vi "Logout_from_webserver_with_idletime.vi"() -> ()   [LabVIEW 2017]
uses:
  Generic_Common/Webserver/html_report_cluster.ctl
  <vilib>/httpClient/LabVIEWHTTPClient.lvlib
panel:
  out "idle_time":string
  out "StatusCodeName":string
  out "Session id name":string
  out "logout_url":string
  out "ErrorCode_expected":string
  out "Logout : Header  debug purpose":string
  out "Logout : Body debug purpose":string
  out "Status_message":string
  out "Logo":u16(ring)
  out "Iteration_Indicator":dbl
  out "Error code recieved":i32
  out "POST_command":string
  out "Command_url":string
  out "Test case":string
  out "Global ini path":path
  out "Test status":picture
  out "Time elapsed for each iteration":string
  out "DelayBetweenIterations":string
  out "Total_Iterations":i32
  out "Global_Webserver_Report":string
  out "TestSuite":string
  out "Error Out":errorcluster
  out "Response time":u32[](graph)
  out "Header of reponse for debug pupose":string
  out "Response from the web server":string
  # "AUTOMATION TESTING WEB SERVICES"
  # "TESTING DETAILS FROM INI"
  # "RESPONSE FROM WEBSERVER"
  # "ms"
  # "Webserver \n1. Webserver is being tested in this test case where SC board of ultrasonic welding machine is connected to test PC \t\t  \nSC IP address: 192.168.2.101, url=https://192.168.2.101\t\t\t\t\t\t\t\t\t\t \t\t\t  \n2. Ports used on SC board are as below:\t\t\t\t\t\t\t\t\t\t\t\t\t\t\t\t\t\t\t\t\t  \n   - J103: (Ethernet0) This port connected to UI controller large screen HMI display\trestricted webservices in this port\t\t\t\t\t\t\t\t\t  \n  - J104: (Ethernet1) This port is connected to local area network for accessing the webpage and testing  webserver                                \n  - J112: SC Logs are taken from this port. TeraTerm is configured  to this port so that SC logs are displayed on the screen."
  # "ms"
  # "Debug purpose"
  # "RESPONSE TIME GRAPH"
  # "TESTING STATUS"
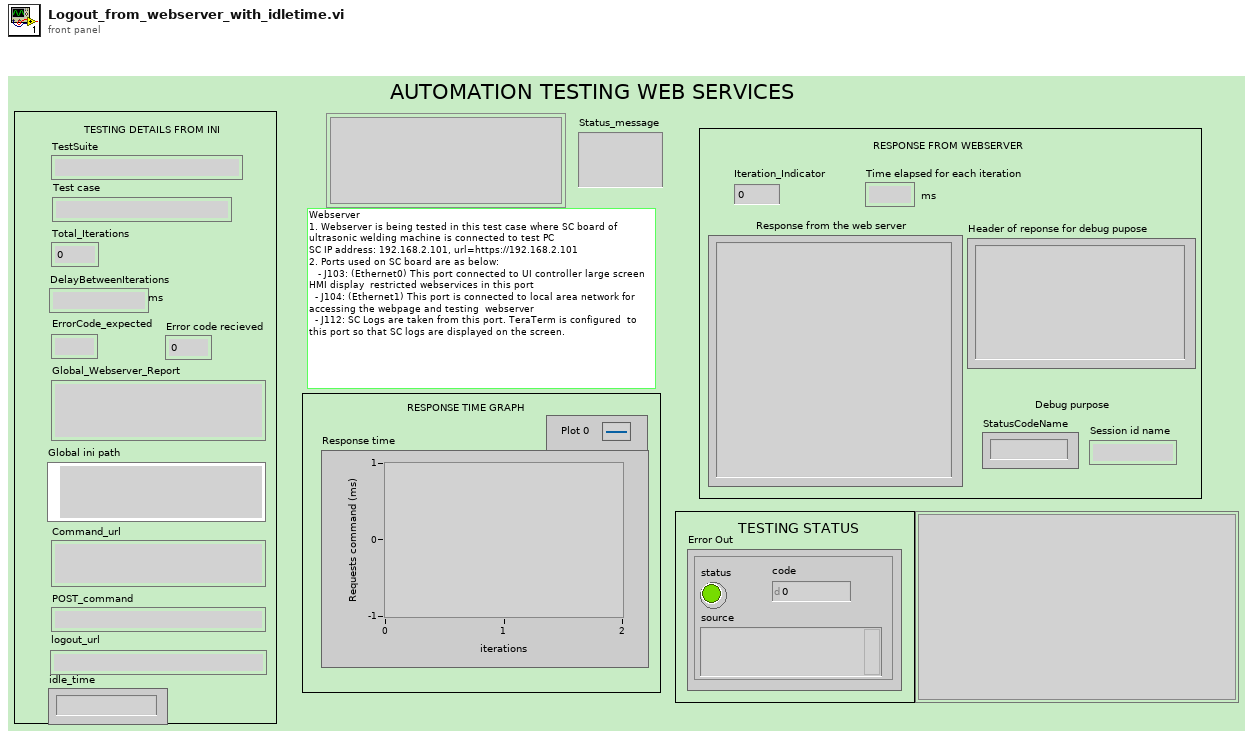
[diagram p1: front panel]
types:
  T1 = enum16{"open", "replace", "create", "open or create", "replace or create", "replace or create with confirmation"}
  T2 = enum8{"Enabled", "Disabled", "Disabled and Grayed Out"}
  T3 = cluster{"[0]":string, "[1]":string, "[2]":string, "[3]":string, "[4]":string, "[5]":string, "[6]":string, "[7]":string, "[8]":string}
  T4 = cluster{"login_url":string, "userid":string, "password":string, "idle_time":string, "command_url":string, "POST_command":string, "StatusCode_expected":string, "Iterations":string, "DelayBetweenIterations":string, "Timeout":string, "logout_url":string, "TestSuite":string, "key":string}
  T5 = cluster{"Server_IP_Address":string, "Server_Port_Number":string, "Sid":string, "StatusCodeName":string, "Global_Webserver_Report":string}
  T6 = typedef "html_report_cluster.ctl" = cluster{"Remarks":string, "Verdict":string, "Status Code":i32, "Status Description":string, "JazzDashboardLink":string, "ReprtPath":string, "Timestamp":string, "TestSuite":string, "TestCase":string, "Iterations":i64, "Time taken to execute  test in msec":string, "Delay Between Iterations":i64}
  T7 = typedef "LabVIEWHTTPClient.lvlib/ClientHandle.ctl" = refnum<k1>
  T8 = typedef "imagedata.ctl" = cluster{"image type":i32, "image depth":i32, "image":u8[], "mask":u8[], "colors":u32[], "Rectangle":cluster{"left":i16, "top":i16, "right":i16, "bottom":i16}}
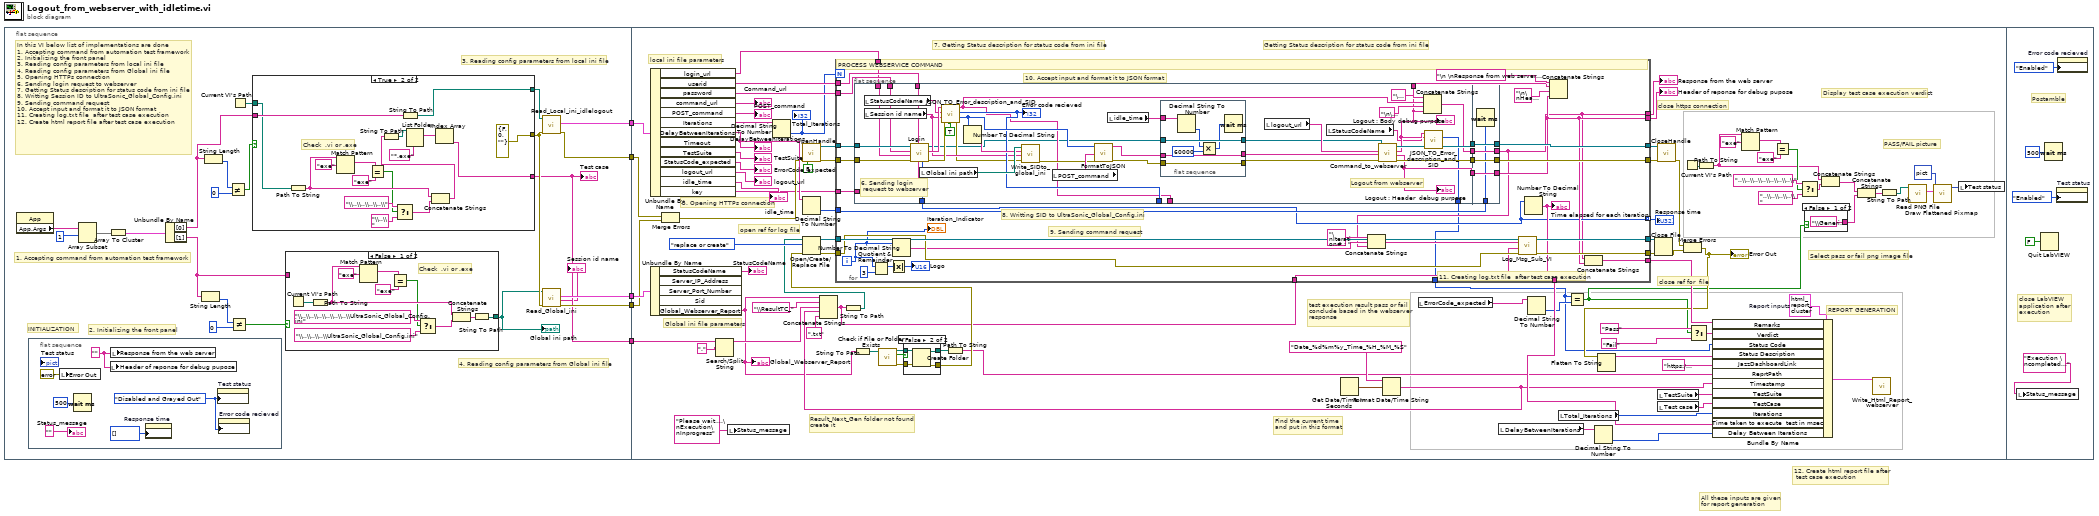
[diagram p0: block diagram]
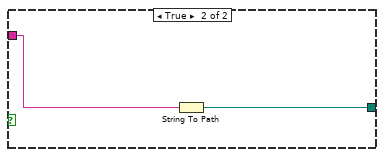
[diagram p2: hidden frame]
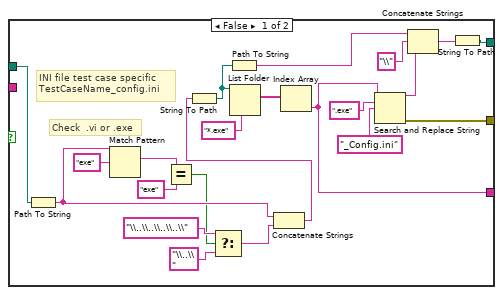
[diagram p3: hidden frame]
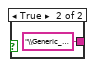
[diagram p5: hidden frame]
diagram:
  # "All these inputs are given \nfor report generation"
  # "12. Create html report file after\n test case execution"
  n1 = flat-sequence {
    tunnel: [w16] -> w5
    tunnel: [w19] -> w4
    tunnel: [w18] -> w3
    tunnel: [w17] -> w2
    tunnel: [w7] -> w1
    tunnel: w5 -> [w141]
    tunnel: w4 -> [w173]
    tunnel: w3 -> [w174]
    tunnel: w2 -> [w140]
    tunnel: w1 -> [w113]
    frame #0 {
      # "INITIALIZATION"
      # "4. Reading config parameters from Global ini file"
      # "3. Reading config parameters from local ini file"
      # "2. Initializing the front panel"
      # "1. Accepting command from automation test framework"
      # "In this VI below list of implementations are done\n1. Accepting command from automation test framework\n2. Initializing the front panel\n3. Reading config parameters from local ini file\n4. Reading config parameters from Global ini file\n5. Opening HTTPs connection\n6. Sending login request to webserver\n7. Getting Status description for status code from ini file\n8. Writting Session ID to UltraSonic_Global_Config.ini\n9. Sending command request\n10. Accept input and format it to JSON format\n11. Creating log.txt file  after test case execution\n12. Create html report file after test case execution"
      n2 = property class="App"() -> ("App.Args"=w21:string[])  [unwired: 2 in, 2 out]
      n3 = flat-sequence {
        frame #0 {
          w28 = T2."Disabled and Grayed Out" ("Disabled")
          w33 = ""
          n4 = local write "Error Out"(errorcluster {"status"=FALSE, "code"=0, "source"=""} ("error constant")) -> ()
          n5 = Wait (ms)(milliseconds to wait=u32 500) -> ()  [unwired: 1 out]
          n6 = local write "Header of reponse for debug pupose"(w33) -> ()
          n7 = local write "Response from the web server"(w33) -> ()
          n8 = property on="Response time" class="WFChart (strict)"("History Data"=u32[] []) -> ()  [unwired: 2 in, 2 out]
          n9 = property on="Test status" class="Pict"("DisabledEnum"=w28) -> ()  [unwired: 2 in, 2 out]
          n10 = property on="Error code recieved" class="DigNum (strict)"("DisabledEnum"=w28) -> ()  [unwired: 2 in, 2 out]
          "Status_message" <- ""
        }
      }
      n11 = Array Subset "Array Subset"(array=w21, index=1) -> (w22:string[])  [unwired: 1 in]
      n12 = Array To Cluster(array=w22) -> (cluster=w23:T3)
      n13 = Unbundle By Name "Unbundle By Name"(w23) -> ("[0]"=w15:string, "[1]"=w10:string)
      n14 = String Length(string=w10) -> (length=w27:i32)
      n15 = String Length(string=w15) -> (length=w24:i32)
      n16 = Not Equal?(x=w24, y=0) -> (x != y?=w13:bool)
      n17 = Not Equal?(x=w27, y=0) -> (x != y?=w11:bool)
      n18 = Current VI's Path() -> (path=w14:path)
      n19 = case shown="True" w13 {
        tunnel: w15 -> [_ w85]
        tunnel: [w61 w84] -> w8
        tunnel: [w60 errorcluster {"status"=FALSE, "code"=0, "source"=""} ("error out")] -> w12
        tunnel: w14 -> [w49 w70]
        tunnel: [w47 w69] -> w7
        frame False {
          # "Check  .vi or .exe"
          # "INI file test case specific\nTestCaseName_config.ini"
          n20 = Path To String(path=w49) -> (string=w54:string)
          n21 = Match Pattern(string=w54, regular expression="exe") -> (match substring=w53:string)  [unwired: 1 in, 3 out]
          n22 = Equal?(x=w53, y="exe") -> (x = y?=w51:bool)
          n23 = Select(t="\\..\\..\\..\\..\\" ("string"), s=w51, f="\\..\\" ("string")) -> (s? t:f=w55:string)
          n24 = Concatenate Strings(w54, w55) -> (w48:string)
          n25 = String To Path(string=w48) -> (path=w59:path)
          n26 = Path To String(path=w59) -> (string=w58:string)
          n27 = List Folder(path=w59, pattern="*.exe") -> (filenames=w62:string[])  [unwired: 2 in, 3 out]
          n28 = Index Array(array=w62) -> (element=w47:string)  [unwired: 1 in]
          n29 = Search and Replace String(input string=w47, search string=".exe", replace string="_Config.ini" ("replace string (\"\")")) -> (result string=w66:string, error out=w60:errorcluster)  [unwired: 5 in, 2 out]
          n30 = Concatenate Strings(w58, "\\" ("string"), w66) -> (w64:string)
          n31 = String To Path(string=w64) -> (path=w61:path)
        }
        frame True {
          # "Check  .vi or .exe"
          n32 = Path To String(path=w70) -> (string=w76:string)
          n33 = Match Pattern(string=w76, regular expression="exe") -> (match substring=w75:string)  [unwired: 1 in, 3 out]
          n34 = Equal?(x=w75, y="exe") -> (x = y?=w73:bool)
          n35 = Select(t="\\..\\..\\..\\..\\" ("string"), s=w73, f="\\..\\" ("string")) -> (s? t:f=w77:string)
          n36 = String To Path(string=w85) -> (path=w84:path)
          n37 = Concatenate Strings(w76, w77) -> (w71:string)
          n38 = String To Path(string=w71) -> (path=w80:path)
          n39 = List Folder(path=w80, pattern="*.exe") -> (filenames=w81:string[])  [unwired: 2 in, 3 out]
          n40 = Index Array(array=w81) -> (element=w69:string)  [unwired: 1 in]
        }
      }
      "Test case" <- w7
      n41 = case shown="False" w11 {
        tunnel: [w43 w46] -> w9
        tunnel: w10 -> [_ w45]
        frame False {
          # "Check  .vi or .exe"
          n42 = Current VI's Path() -> (path=w35:path)
          n43 = Path To String(path=w35) -> (string=w39:string)
          n44 = Match Pattern(string=w39, regular expression="exe") -> (match substring=w38:string)  [unwired: 1 in, 3 out]
          n45 = Equal?(x=w38, y="exe") -> (x = y?=w36:bool)
          n46 = Select(t="\\..\\..\\..\\..\\..\\..\\UltraSonic_Global_Config.ini" ("string"), s=w36, f="\\..\\..\\..\\UltraSonic_Global_Config.ini" ("string")) -> (s? t:f=w40:string)
          n47 = Concatenate Strings(w39, w40) -> (w44:string)
          n48 = String To Path(string=w44) -> (path=w43:path)
        }
        frame True {
          n49 = String To Path(string=w45) -> (path=w46:path)
        }
      }
      "Global ini path" <- w9
      n50 = call "Read_Local_ini_idlelogout.vi"("Error In"=w12, "Local ini path"=w8) -> ("Error Out"=w16:errorcluster, "Read from ini file"=w18:T4)  [unwired: 8 in]
      n51 = call "Read_Global_ini.vi"("Error In"=w12, "Global ini path"=w9) -> ("Error Out"=w17:errorcluster, "Session id name"=→"Session id name":string, "Global Cluster"=w19:T5)  [unwired: 7 in]
    }
    frame #1 {
      w156 = T6 {"Remarks"="", "Verdict"="", "Status Code"=0, "Status Description"="", "JazzDashboardLink"="", "ReprtPath"="", "Timestamp"="", "TestSuite"="", "TestCase"="", "Iterations"=0, "Time taken to execute  test in msec"="", "Delay Between Iterations"=1000}  # Report inputs
      # "Getting Status description for status code from ini file"
      # "7. Getting Status description for status code from ini file"
      # "Select pass or fail png image file"
      # "test execution result pass or fail\nconclude based in the webserver\nresponse"
      # "Find the current time \nand put in this format"
      # "open ref for log file"
      # "Result_Next_Gen folder not found\ncreate it"
      # "Global ini file parameters"
      # "local ini file parameters"
      # "close ref for  file"
      # "close https connection"
      # "Display test case execution verdict"
      # "11. Creating log.txt file  after test case execution"
      # "5. Opening HTTPs connection"
      # "REPORT GENERATION"
      # "PASS/FAIL picture"
      n52 = Unbundle By Name(w173) -> ("StatusCodeName"=→"StatusCodeName":string, "Global_Webserver_Report"=w105:string)  [unwired: 3 out]
      "Global_Webserver_Report" <- w105
      n53 = Unbundle By Name(w174) -> ("login_url"=w136:string, "userid"=w170:string, "password"=w169:string, "command_url"=→"Command_url":string, "POST_command"=→"POST_command":string, "Iterations"=w166:string, "DelayBetweenIterations"=w165:string, "TestSuite"=→"TestSuite":string, "StatusCode_expected"=→"ErrorCode_expected":string, "logout_url"=→"logout_url":string, "idle_time"=→"idle_time":string, "key"=w86:string)  [unwired: 1 out]
      "DelayBetweenIterations" <- w165
      n54 = Merge Errors(w141, w140) -> (w139:errorcluster)
      n55 = Search/Split String(string=w113, search string/char (-)=".") -> (substring before match=w111:string)  [unwired: 1 in, 2 out]
      n56 = local write "Status_message"("Please wait....\nExecution\nInprogress") -> ()
      n57 = Decimal String To Number(string=w166) -> (number=w154:i32)  [unwired: 2 in, 1 out]
      "Total_Iterations" <- w154
      n58 = call <vilib>:"OpenHandle.vi"("error in (no error)"=w139, "verify server(true)"=FALSE) -> ("client handle out"=w172:T7, "error out"=w171:errorcluster)  [unwired: 12 in]
      n59 = Decimal String To Number(string=w165) -> (number=w164:i32)  [unwired: 2 in, 1 out]
      n60 = String To Path(string=w105) -> (path=w110:path)
      n61 = call <vilib>:"Check if File or Folder Exists.vi"("path"=w110) -> ("error out"=w106:errorcluster, "file or folder exists?"=w109:bool, "dup path"=w108:path)  [unwired: 8 in]
      n62 = case shown="False" w109 {
        tunnel: [w175 w180] -> w104
        tunnel: w108 -> [w176 w179]
        tunnel: [w176 w178] -> w107
        tunnel: w106 -> [w175 w177]
        frame True {
        }
        frame False {
          n63 = Create Folder(path (use dialog)=w179, error in=w177) -> (created path=w178:path, error out=w180:errorcluster)  [unwired: 1 in, 1 out]
        }
      }
      n64 = Path To String(path=w107) -> (string=w103:string)
      n65 = Get Date/Time In Seconds() -> (seconds since 1Jan1904=w92:timestamp)
      n66 = Format Date/Time String(time format string (%c)="Date_%d%m%y_Time_%H_%M_%S", seconds (now)=w92) -> (date/time string=w116:string)  [unwired: 1 in]
      n67 = Concatenate Strings(w105, "\\ResultTC_" ("string"), w111, w116, ".txt" ("string")) -> (w91:string)
      n68 = String To Path(string=w91) -> (path=w114:path)
      n69 = Open/Create/Replace File(file path (use dialog)=w114, error in=w104, operation (0:open)=T1."replace or create") -> (refnum out=w163:refnum<file>, error out=w162:errorcluster)  [unwired: 3 in, 1 out]
      n70 = for {
        N: w154 -> [_]
        tunnel: w172 -> [w216]
        tunnel: w169 -> [w213]
        tunnel: [w185] -> w168
        tunnel: w170 -> [w214]
        tunnel: [w198] -> w167
        tunnel: w171 -> [w215]
        tunnel: w164 -> [w192]
        tunnel: [w186] -> w147 mode=indexing
        tunnel: w163 -> [w211]
        tunnel: w162 -> [w210]
        tunnel: [w209] -> w161
        tunnel: [w208] -> w160
        tunnel: [w204] -> w158
        tunnel: [w203] -> w157
        tunnel: [w199] -> w145
        tunnel: w136 -> [w201]
        tunnel: [w197] -> w118
        tunnel: w91 -> [w187]
        tunnel: [w184] -> w87
        tunnel: w86 -> [w183]
        i -> [w194]
        # "8. Writting SID to UltraSonic_Global_Config.ini"
        # "10. Accept input and format it to JSON format"
        # "9. Sending command request"
        # "PROCESS WEBSERVICE COMMAND"
        n71 = flat-sequence {
          tunnel: w214 -> [w251]
          tunnel: w213 -> [w250]
          tunnel: [w237] -> w191
          tunnel: [w236] -> w190
          tunnel: [w247] -> w189
          tunnel: [w246] -> w188
          tunnel: w201 -> [w249]
          tunnel: [w220] -> w200
          tunnel: [w235] -> _
          tunnel: [w231] -> _
          tunnel: [w240] -> w186
          tunnel: w216 -> [w253]
          tunnel: w215 -> [w252]
          tunnel: [w218] -> w184
          tunnel: w183 -> [w217]
          tunnel: [w262] -> w203
          tunnel: [w263] -> w204
          tunnel: [w264] -> w198
          tunnel: [w265] -> w185
          tunnel: w191 -> [w265]
          tunnel: w190 -> [w264]
          tunnel: w189 -> [w263]
          tunnel: w188 -> [w262]
          tunnel: w192 -> [w261]
          frame #0 {
            # "Logout from webserver"
            # "6. Sending login\n request to webserver"
            n72 = local read "StatusCodeName"() -> (w233:string)
            n73 = local read "Session id name"() -> (w232:string)
            n74 = call "Login.vi"("key"=w217, "userid"=w251, "Error In"=w252, "Command to webservice"=w249, "password"=w250, "IN HTTPS client handle"=w253) -> ("Error Out"=w242:errorcluster, "Body of reponse"=w239:string, "OUT HTTPS client handle"=w223:T7, "Response time"=w240:u32)  [unwired: 1 in, 1 out]
            n75 = local read "Global ini path"() -> (w245:path)
            n76 = call "JSON_TO_Error_description_and_SID.vi"("Sid_present_in_webserver_response"=TRUE, "Error In"=w242, "Session id name"=w232, "Status code name"=w233, "JSON String input"=w239) -> ("Error Out"=w228:errorcluster, "SID"=w238:i32, "status code"=w235:i32, "status_selected"=w231:string)  [unwired: 3 in]
            "Error code recieved" <- w235
            n77 = Number To Decimal String(number=w238) -> (decimal integer string=w243:string)  [unwired: 1 in]
            n78 = call "Write_SIDto_global_ini.vi"("Error In"=w228, "Session id name"=w232, "SID"=w243, "Global ini path"=w245) -> ("Error Out"=w244:errorcluster)  [unwired: 7 in]
            n79 = local read "POST_command"() -> (w248:string)
            n80 = call "FormatToJSON.vi"("Error In"=w244, "Post_command"=w248, "Sid"=w238) -> ("Error Out"=w225:errorcluster, "Final_POST_Command"=w227:string)  [unwired: 6 in, 1 out]
            n81 = local read "idle_time"() -> (w221:string)
            n82 = flat-sequence {
              tunnel: w227 -> [w260]
              tunnel: [w260] -> w226
              tunnel: w225 -> [w259]
              tunnel: [w259] -> w224
              tunnel: w223 -> [w258]
              tunnel: [w258] -> w222
              tunnel: w221 -> [w257]
              frame #0 {
                n83 = Decimal String To Number(string=w257) -> (number=w256:i32)  [unwired: 2 in, 1 out]
                n84 = Multiply(x=w256, y=60000) -> (x*y=w254:i32)
                n85 = Wait (ms)(milliseconds to wait=w254) -> ()  [unwired: 1 out]
              }
            }
            n86 = local read "logout_url"() -> (w241:string)
            n87 = local read "StatusCodeName"() -> (w219:string)
            n88 = call "Command_to_webserver.vi"("Error In"=w224, "JSON post command"=w226, "URL Command to Logout"=w241, "https client handle in ref"=w222) -> ("Error Out"=w247:errorcluster, "Header of response for debug purpose"=w236:string, "Body of response"=w220:string, "https client handle out ref"=w246:T7)  [unwired: 3 in, 1 out]
            "Logout : Body debug purpose" <- w220
            "Logout : Header  debug purpose" <- w236
            n89 = Concatenate Strings("\nLogin:\n" ("string"), w231, "\n\nLogout:\n" ("string"), w220) -> (w237:string)
            n90 = call "JSON_TO_Error_description_and_SID.vi"("Status code name"=w219, "JSON String input"=w220) -> ("status code"=w218:i32)  [unwired: 6 in, 3 out]
          }
          frame #1 {
            n91 = Wait (ms)(milliseconds to wait=w261) -> ()  [unwired: 1 out]
          }
        }
        n92 = Quotient & Remainder(x=w194, y=3) -> (x-y*floor(x/y)=w195:i32)  [unwired: 1 out]
        n93 = Absolute Value(x=w195) -> (abs(x)=→"Logo":i32)
        n94 = Number To Decimal String(number=w194) -> (decimal integer string=w205:string)  [unwired: 1 in]
        n95 = Concatenate Strings("\nIteration# : " ("string"), w205, w185) -> (w207:string)
        n96 = call "Log_Msg_Sub_VI.vi"("Error In"=w210, "Path for CSV"=w187, "String input"=w207, "refnum in"=w211) -> ("Error Out"=w208:errorcluster, "refnum out"=w209:refnum<file>)  [unwired: 6 in]
        n97 = Number To Decimal String(number=w186) -> (decimal integer string=w197:string)  [unwired: 1 in]
        "Time elapsed for each iteration" <- w197
        n98 = Concatenate Strings("\n \nResponse from web server# :\n" ("string"), w200, "\n\nHeader# : \n", w198) -> ()  [unwired: 1 out]
        n99 = Concatenate Strings(w185, w198) -> (w199:string)
        "Iteration_Indicator" <- w194
      }
      "Response from the web server" <- w168
      "Header of reponse for debug pupose" <- w167
      "Response time" <- w147
      n100 = local read "ErrorCode_expected"() -> (w97:string)
      n101 = local read "DelayBetweenIterations"() -> (w149:string)
      n102 = Decimal String To Number(string=w97) -> (number=w96:i32)  [unwired: 2 in, 1 out]
      n103 = local read "Total_Iterations"() -> (w150:i32)
      n104 = Equal?(x=w87, y=w96) -> (x = y?=w95:bool)
      n105 = Decimal String To Number(string=w149) -> (number=w148:i32)  [unwired: 2 in, 1 out]
      n106 = Close File(refnum=w161, error in=w160) -> (error out=w152:errorcluster)  [unwired: 1 out]
      n107 = call <vilib>:"CloseHandle.vi"("client handle"=w157, "error in (no error)"=w158) -> ("error out"=w153:errorcluster)  [unwired: 13 in]
      n108 = local read "TestSuite"() -> (w151:string)
      n109 = local read "Test case"() -> (w138:string)
      n110 = Current VI's Path() -> (path=w124:path)
      n111 = Merge Errors(w153, w152) -> (w102:errorcluster)
      "Error Out" <- w102
      n112 = Flatten To String(anything=w102) -> (data string=w101:string)  [unwired: 3 in, 2 out]
      n113 = Select(t="Pass", s=w95, f="Fail") -> (s? t:f=w142:string)
      n114 = Path To String(path=w124) -> (string=w122:string)
      n115 = Bundle By Name(cluster=w156, "Remarks"=w145, "Verdict"=w142, "Status Code"=w87, "Status Description"=w101, "JazzDashboardLink"="https://jazz.bucclm.com/", "ReprtPath"=w103, "Timestamp"=w116, "TestSuite"=w151, "TestCase"=w138, "Iterations"=w150, "Time taken to execute  test in msec"=w118, "Delay Between Iterations"=w148) -> (w155:T6)
      n116 = Match Pattern(string=w122, regular expression="exe") -> (match substring=w128:string)  [unwired: 1 in, 3 out]
      n117 = Equal?(x=w128, y="exe") -> (x = y?=w126:bool)
      n118 = Select(t="..\\..\\..\\..\\..\\..\\..\\" ("string"), s=w126, f="..\\..\\..\\..\\" ("string")) -> (s? t:f=w123:string)
      n119 = case shown="False" w95 {
        tunnel: ["\\Generic_Common\\\\Webserver\\\\Fail.png" "\\Generic_Common\\\\Webserver\\\\Pass.png"] -> w132
        frame False {
        }
        frame True {
        }
      }
      n120 = Concatenate Strings(w122, w123) -> (w121:string)
      n121 = Concatenate Strings(w121, w132) -> (w131:string)
      n122 = call "Write_Html_Report_webserver.vi"("Report inputs"=w155) -> ()  [unwired: 18 in, 1 out]
      n123 = String To Path(string=w131) -> (path=w120:path)
      n124 = call <vilib>:"Read PNG File.vi"("path to PNG file"=w120) -> ("image data"=w119:T8)  [unwired: 8 in, 2 out]
      n125 = call <vilib>:"Draw Flattened Pixmap.vi"("image data"=w119, "picture"=picture data[5B]) -> ("new picture"=w90:picture)  [unwired: 7 in]
      n126 = local write "Test status"(w90) -> ()
    }
    frame #2 {
      # "close LabVIEW \napplication after \nexecution"
      # "Postamble"
      n127 = local write "Status_message"("Execution \ncompleted...") -> ()
      n128 = Quit LabVIEW(quit? (T)=FALSE) -> ()
      n129 = Wait (ms)(milliseconds to wait=u32 500) -> ()  [unwired: 1 out]
      n130 = property on="Test status" class="Pict"("DisabledEnum"=T2."Enabled" ("Disabled")) -> ()  [unwired: 2 in, 2 out]
      n131 = property on="Error code recieved" class="DigNum (strict)"("DisabledEnum"=T2."Enabled" ("Disabled")) -> ()  [unwired: 2 in, 2 out]
    }
  }
